vi "Convert Vector 3D (SGL) To Point 2D (SGL).vi"(11 "Vector 3D":T2) -> (3 "Point 2D":T1)   [LabVIEW 2022 SP3, in "3D.lvlib"]
uses:
  3D.lvlib
  Point 2D.ctl
  Vector 3D.ctl
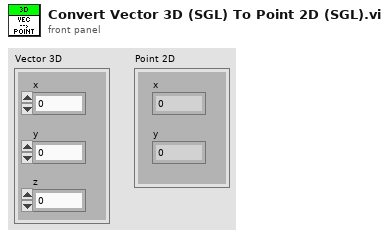
[diagram p1: front panel]
types:
  T1 = typedef "3D.lvlib/Point 2D.ctl" = cluster{"x":sgl, "y":sgl}
  T2 = typedef "3D.lvlib/Vector 3D.ctl" = cluster{"x":sgl, "y":sgl, "z":sgl}
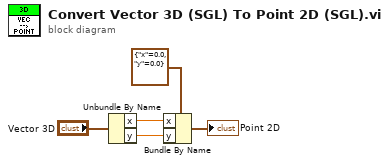
[diagram p0: block diagram]
diagram:
  n1 = Unbundle By Name("Vector 3D") -> ("x"=w2:sgl, "y"=w1:sgl)
  n2 = Bundle By Name(cluster=T1 {"x"=0.0, "y"=0.0} ("Point 2D"), "x"=w2, "y"=w1) -> (→"Point 2D":T1)
